vi "Get Right Value.vi"(11 "arm.lvclass":refnum<class "arm.lvclass">) -> (2 "Value":dbl, 3 "arm.lvclass":refnum<class "arm.lvclass">)   [LabVIEW 2015, in "arm.lvclass"]
uses:
  arm.lvclass
  arm.lvclass/arm.ctl
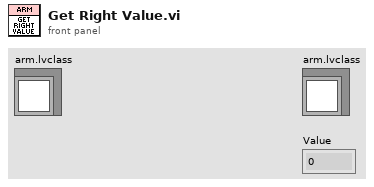
[diagram p1: front panel]
types:
  T1 = typedef "WPI_PotentiometerDevRef.ctl" = cluster{"DevStatus":errorcluster, "Analog Channel":T2, "Invert Output":bool}
  T2 = typedef "FPGA_AIChannel.ctl" = enum8{"AI 0", "AI 1", "AI 2", "AI 3", "AI MXP 0", "AI MXP 1", "AI MXP 2", "AI MXP 3", "Invalid"}
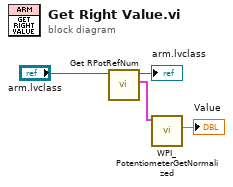
[diagram p0: block diagram]
diagram:
  n1 = call "Get RPotRefNum.vi"("arm in"="arm.lvclass") -> ("PotDevRef"=w3:T1, "arm out"=→"arm.lvclass":refnum<class "arm.lvclass">)  [unwired: 9 in]
  n2 = call <vilib>:"WPI_PotentiometerGetNormalized.vi"("PotDevRef"=w3) -> ("Normalized Value"=→"Value":dbl)  [unwired: 8 in, 2 out]
